vi "KeyBoardSimulation.vi"(0 "VI Reference In":refnum<vi>, 5 "Control Path":string, 7 "Key Array":T1(array[cluster])=[{" Key"=16, "Action"=enum."Down", "Delay (ms)"=10}, {" Key"=72, "Action"=enum."Press", "Delay (ms)"=100}, {" Key"=16, "Action"=enum."Up", "Delay (ms)"=10}, {" Key"=69, "Action"=enum."Press", "Delay (ms)"=100}, {" Key"=76, "Action"=enum."Press", "Delay (ms)"=100}, {" Key"=76, "Action"=enum."Press", "Delay (ms)"=100}, {" Key"=79, "Action"=enum."Press", "Delay (ms)"=100}], 11 "error In":errorcluster) -> (4 "VI Reference Out":refnum<vi>, 15 "error IO":errorcluster)   [LabVIEW 2016, in "Drona.lvlib"]
doc: "Uses simulated Key Presses to type into a String/Numeric control programmatically."
uses:
  Drona.lvlib
  Setup/GetControlRef/GetControlRefByPath.vi
  Setup/GetControlRef/GetControlRef.lvlib
panel:
  # "Overview: This VI is an example that uses simulated Key Presses to type into a String control programmatically.  \n\nInstructions:\n1. Enter the keys in the Key Array control. It is what defines which keys are pressed and for how long.  Note that the shift key is pushed down and up in separate steps and that the alphabetical keys are pressed. This is equivalent to holding the shift key down while pressing\n'H', the result being an uppercase 'H'.\n2. Run this VI and 'Hello' will be programmatically typed in the Output box."
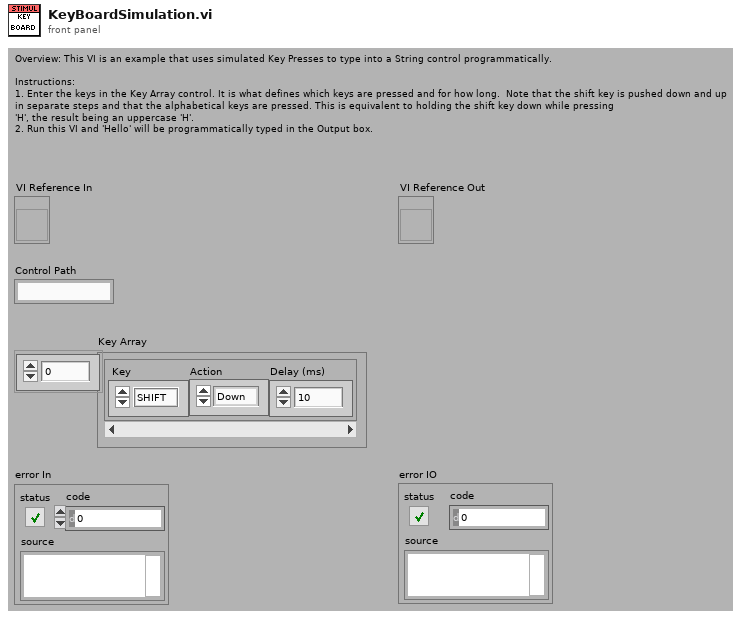
[diagram p1: front panel]
types:
  T1 = cluster{" Key":u8, "Action":enum16{"Press", "Up", "Down"}, "Delay (ms)":u32}[]
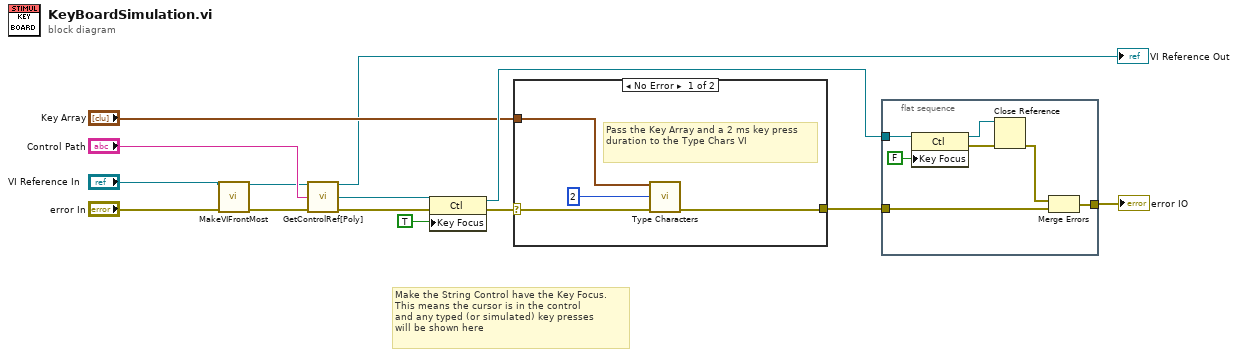
[diagram p0: block diagram]
diagram:
  # "Make the String Control have the Key Focus.\nThis means the cursor is in the control\nand any typed (or simulated) key presses\nwill be shown here"
  n1 = call "MakeVIFrontMost.vi"("VI Reference In"="VI Reference In", "error in"="error In") -> ("VI Reference Out"=w1:refnum<vi>, "error out"=w4:errorcluster)  [unwired: 12 in]
  n2 = call-poly "GetControlRef[Poly].vi"("VI Reference In"=w1, "Control Path"="Control Path", "error In"=w4) -> ("VI Reference Out"=→"VI Reference Out":refnum<vi>, "Ctl Refnum"=w6:refnum<vi>, "error out"=w13:errorcluster)  [unwired: 10 in]
  n3 = property class="Ctl"(reference=w6, error in=w13, "Key Focus"=TRUE) -> (reference out=w10:refnum<vi>, error out=w12:errorcluster)
  n4 = case shown="No Error" w12 {
    selector: w12 -> [w16 w19]
    tunnel: [w15 w19] -> w11
    tunnel: "Key Array" -> [w18 _]
    frame No Error {
      # "Pass the Key Array and a 2 ms key press\nduration to the Type Chars VI"
      n5 = call "Type Characters.vi"("Key Array"=w18, "Length of Key Press (ms)"=u32 2, "error in"=w16) -> ("error out"=w15:errorcluster)  [unwired: 12 in]
    }
    frame Error {
    }
  }
  n6 = flat-sequence {
    tunnel: w11 -> [w26]
    tunnel: w10 -> [w24]
    tunnel: [w22] -> w9
    frame #0 {
      n7 = property class="Ctl"(reference=w24, "Key Focus"=FALSE) -> (reference out=w20:refnum<vi>, error out=w25:errorcluster)  [unwired: 1 in]
      n8 = Close Reference(reference=w20, error in (no error)=w25) -> (error out=w21:errorcluster)
      n9 = Merge Errors(w21, w26) -> (w22:errorcluster)
    }
  }
  "error IO" <- w9
